vi "process_stim_NI.vi"(8 "error in (no error)":errorcluster) -> (0 "error out":errorcluster)   [LabVIEW 2010]
uses:
  typedefs/control_stim_enum.ctl
  typedefs/run_mode.ctl
  typedefs/device_parameters.ctl
  typedefs/protocol_parameters.ctl
  typedefs/free_run_parameters.ctl
  <vilib>/DAQmx/write.llb/DAQmx Write (Analog 1D DBL 1Chan NSamp).vi
  <vilib>/daqmx/miscellaneous.llb/DAQmx Fill In Error Info.vi
  Program Files/National Instruments/LabVIEW 2010/resource/objmgr/daqmx.rc
panel:
  out "Time [s]":dbl caption="[s]"
  out "Protocol":dbl[](graph)
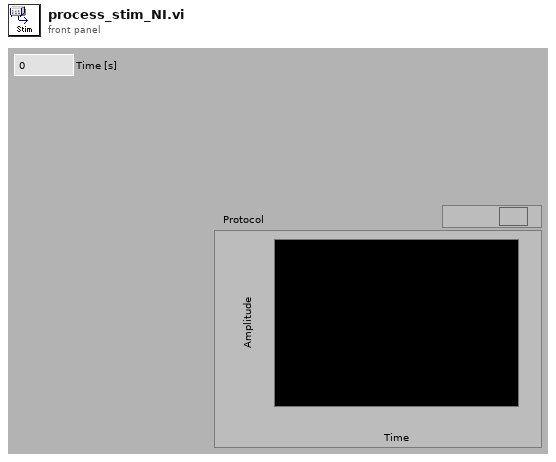
[diagram p1: front panel]
types:
  T1 = typedef "control_stim_enum.ctl" = enum16{"Init", "Stim Protocol", "Stim Free Run", "Stop", "Quit"}
  T2 = cluster{"Control stim Enum":T1, "variant":variant}
  T3 = typedef "run_mode.ctl" = enum32{"Protocol", "Free Run"}
  T4 = typedef "device_parameters.ctl" = cluster{"Triggered?":bool, "Shutter channel":tag, "Acquisition channels":tag, "Acquisition sample rate":dbl, "Read chunk size":i32, "Stimulation channel":tag, "Stimulation sample rate":dbl}
  T5 = typedef "protocol_parameters.ctl" = cluster{"Repetitions":dbl, "ON time":dbl, "OFF time":dbl, "Stim onset":dbl, "Stim frequency":dbl, "Pulse width":dbl, "Acquire before ON":dbl, "Acquire after ON":dbl, "Sync shutter to acquisition":bool}
  T6 = cluster{"Device parameters":T4, "Protocol parameters":T5}
  T7 = typedef "free_run_parameters.ctl" = cluster{"Stim onset":dbl, "Stim frequency":dbl, "Stim length":dbl, "Sync shutter to acquisition":bool}
  T8 = cluster{"Device parameters":T4, "Free run parameters":T7}
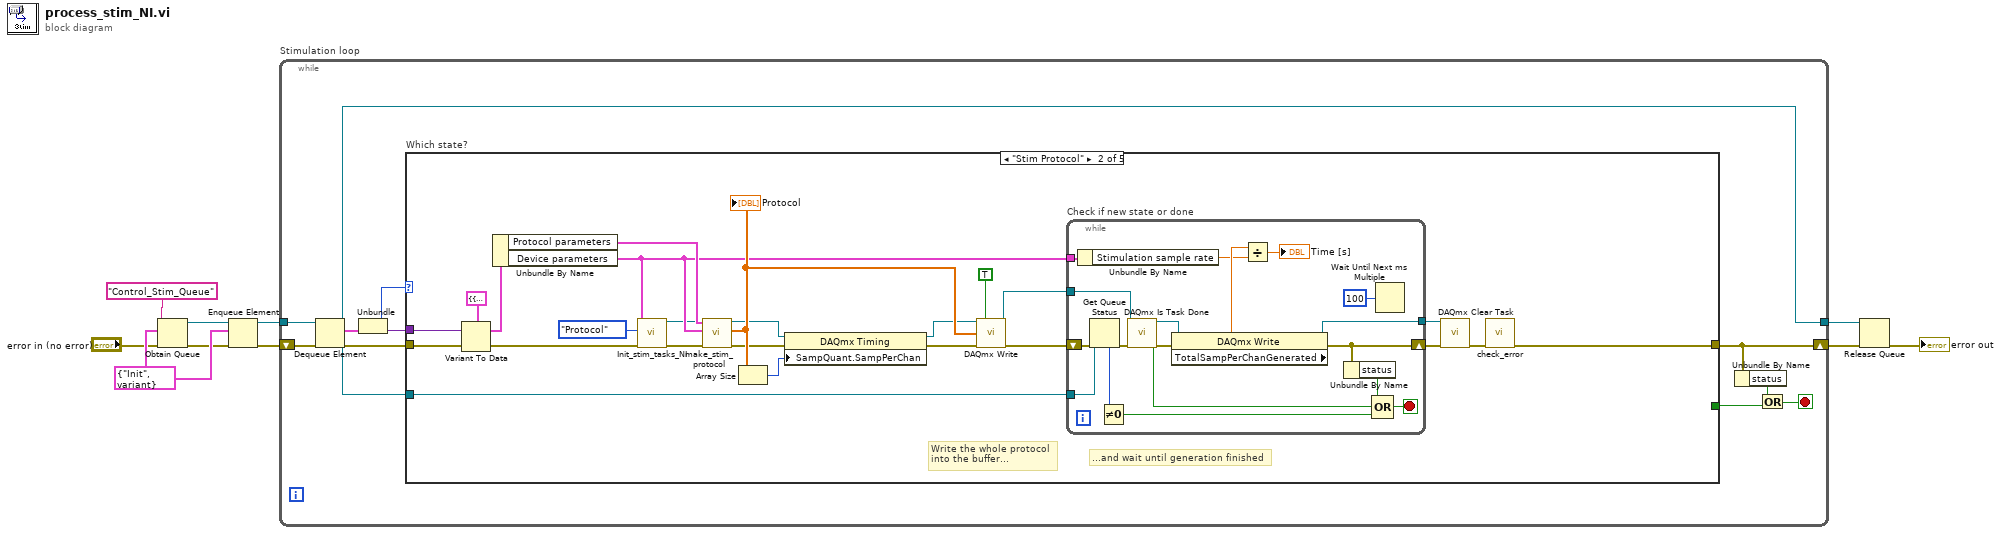
[diagram p0: block diagram]
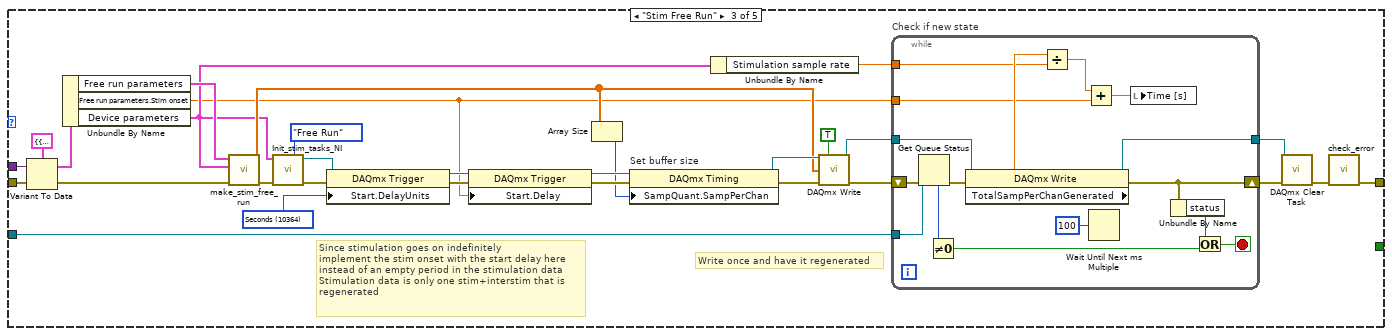
[diagram p3: hidden frame]
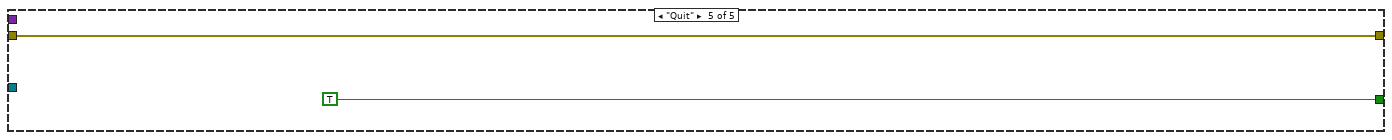
[diagram p5: hidden frame]
diagram:
  w10 = T2 {"Control stim Enum"=enum."Init", "variant"=variant} ("ControlDAQ state cluster")
  n1 = Obtain Queue(name (unnamed)="Control_Stim_Queue", element data type=w10, error in (no error)="error in (no error)") -> (queue out=w6:refnum<queue>, error out=w8:errorcluster)  [unwired: 2 in, 1 out]
  n2 = Enqueue Element(queue=w6, element=w10, error in (no error)=w8) -> (queue out=w7:refnum<queue>, error out=w9:errorcluster)  [unwired: 1 in, 1 out]
  n3 = while "Stimulation loop" {
    shift-right: [w15] -> w5
    shift-left: w9 -> [w20]
    tunnel: w7 -> [w21]
    tunnel: [w11] -> w4
    stop <- w13 stop-if-true
    n4 = Dequeue Element(queue=w21, error in (no error)=w20) -> (queue out=w11:refnum<queue>, element=w19:T2, error out=w17:errorcluster)  [unwired: 1 in, 1 out]
    n5 = Unbundle(w19) -> ("Control stim Enum"=w12:T1, "variant"=w18:variant)
    n6 = case "Which state?" shown="\"Stim Protocol\"" w12 {
      tunnel: w11 -> [_ w43 w72 _ _]
      tunnel: w18 -> [_ w45 w92 _ _]
      tunnel: w17 -> [w22 w44 w93 w110 w111]
      tunnel: [w22 w29 w67 w110 w111] -> w15
      tunnel: [_ _ _ _ TRUE] -> w16
      frame "Init", Default {
      }
      frame "Stim Protocol" {
        # "...and wait until generation finished"
        # "Write the whole protocol\ninto the buffer..."
        n7 = Variant To Data(error in=w44, Variant=w45, type=T6 {"Device parameters"={"Triggered?"=FALSE, "Shutter channel"="", "Acquisition channels"="", "Acquisition sample rate"=0.0, "Read chunk size"=0, "Stimulation channel"="", "Stimulation sample rate"=0.0}, "Protocol parameters"={"Repetitions"=0.0, "ON time"=0.0, "OFF time"=0.0, "Stim onset"=0.0, "Stim frequency"=0.0, "Pulse width"=0.0, "Acquire before ON"=0.0, "Acquire after ON"=0.0, "Sync shutter to acquisition"=FALSE}}) -> (error out=w42:errorcluster, data=w39:T6)
        n8 = Unbundle By Name(w39) -> ("Protocol parameters"=w38:T5, "Device parameters"=w28:T4)
        n9 = call "Init_stim_tasks_NI.vi"("error in"=w42, "Run mode"=run_mode."Protocol", "Device parameters"=w28) -> ("error out"=w41:errorcluster, "Stim task out"=w27:refnum<k21>)  [unwired: 5 in]
        n10 = call "make_stim_protocol.vi"("Error in"=w41, "Device parameters"=w28, "Protocol parameters"=w38) -> ("Error out"=w24:errorcluster, "Stim array"=w37:dbl[])  [unwired: 7 in]
        "Protocol" <- w37
        n11 = Array Size(array=w37) -> (size(s)=w23:i32)
        n12 = property class="DAQmx Timing"(reference=w27, error in=w24, "SampQuant.SampPerChan"=w23) -> (reference out=w26:refnum<k21>, error out=w25:errorcluster)
        n13 = call-poly <vilib>:"DAQmx Write.vi"("task/channels in"=w26, "auto start"=TRUE, "data"=w37, "error in"=w25) -> ("task out"=w34:refnum<k21>, "error out"=w35:errorcluster)  [unwired: 9 in, 1 out]
        n14 = while "Check if new state or done" {
          tunnel: w43 -> [w63]
          tunnel: w34 -> [w60]
          tunnel: [w50] -> w33
          shift-right: [w52] -> w32
          shift-left: w35 -> [w62]
          tunnel: w28 -> [w49]
          stop <- w54 stop-if-true
          n15 = Unbundle By Name(w49) -> ("Stimulation sample rate"=w47:dbl)
          n16 = Get Queue Status(queue=w63, error in (no error)=w62) -> (error out=w61:errorcluster, # elements in queue=w59:i32)  [unwired: 1 in, 6 out]
          n17 = Not Equal To 0?(x=w59) -> (x != 0?=w55:bool)
          n18 = call <vilib>:"DAQmx Is Task Done.vi"("task/channels in"=w60, "error in"=w61) -> ("task out"=w51:refnum<k21>, "task done?"=w56:bool, "error out"=w53:errorcluster)  [unwired: 11 in]
          n19 = property class="DAQmx Write"(reference=w51, error in=w53) -> (reference out=w50:refnum<k21>, error out=w52:errorcluster, "TotalSampPerChanGenerated"=w48:dbl)
          n20 = Divide(x=w48, y=w47) -> (x/y=→"Time [s]":dbl)
          n21 = Unbundle By Name(w52) -> ("status"=w57:bool)
          n22 = Compound Arithmetic op=OR(w57, w56, w55) -> (w54:bool)
          n23 = Wait Until Next ms Multiple(millisecond multiple=u32 100) -> ()  [unwired: 1 out]
        }
        n24 = call <vilib>:"DAQmx Clear Task.vi"("task in"=w33, "error in"=w32) -> ("error out"=w30:errorcluster)  [unwired: 13 in]
        n25 = call "check_error.vi"("error in"=w30) -> ("error out"=w29:errorcluster)  [unwired: 10 in]
      }
      frame "Stim Free Run" {
        w87 = 10364 items=["Sample Clock Periods"=10286, "Seconds"=10364, "Ticks"=10304] ("Start.DelayUnits")
        # "Write once and have it regenerated"
        # "Since stimulation goes on indefinitely\nimplement the stim onset with the start delay here\ninstead of an empty period in the stimulation data\nStimulation data is only one stim+interstim that is\nregenerated"
        n26 = Variant To Data(error in=w93, Variant=w92, type=T8 {"Device parameters"={"Triggered?"=FALSE, "Shutter channel"="", "Acquisition channels"="", "Acquisition sample rate"=0.0, "Read chunk size"=0, "Stimulation channel"="", "Stimulation sample rate"=0.0}, "Free run parameters"={"Stim onset"=0.0, "Stim frequency"=0.0, "Stim length"=0.0, "Sync shutter to acquisition"=FALSE}} ("output cluster")) -> (error out=w82:errorcluster, data=w90:T8)
        n27 = Unbundle By Name(w90) -> ("Free run parameters"=w83:T7, "Free run parameters.Stim onset"=w64:dbl, "Device parameters"=w66:T4)
        n28 = call "make_stim_free_run.vi"("error in"=w82, "Device parameters"=w66, "Free run parameters"=w83) -> ("error out"=w81:errorcluster, "Stim array"=w75:dbl[])  [unwired: 7 in]
        n29 = call "Init_stim_tasks_NI.vi"("error in"=w81, "Run mode"=run_mode."Free Run", "Device parameters"=w66) -> ("error out"=w85:errorcluster, "Stim task out"=w84:refnum<k21>)  [unwired: 5 in]
        n30 = property class="DAQmx Trigger"(reference=w84, error in=w85, "Start.DelayUnits"=w87) -> (reference out=w88:refnum<k21>, error out=w89:errorcluster)
        n31 = property class="DAQmx Trigger"(reference=w88, error in=w89, "Start.Delay"=w64) -> (reference out=w79:refnum<k21>, error out=w80:errorcluster)
        n32 = Array Size(array=w75) -> (size(s)=w78:i32)
        n33 = property on="Set buffer size" class="DAQmx Timing"(reference=w79, error in=w80, "SampQuant.SampPerChan"=w78) -> (reference out=w76:refnum<k21>, error out=w77:errorcluster)
        n34 = Unbundle By Name(w66) -> ("Stimulation sample rate"=w65:dbl)
        n35 = call-poly <vilib>:"DAQmx Write.vi"("task/channels in"=w76, "auto start"=TRUE, "data"=w75, "error in"=w77) -> ("task out"=w69:refnum<k21>, "error out"=w73:errorcluster)  [unwired: 9 in, 1 out]
        n36 = while "Check if new state" {
          tunnel: w72 -> [w108]
          shift-right: [w101] -> w71
          shift-left: w73 -> [w109]
          tunnel: w69 -> [w98]
          tunnel: [w97] -> w70
          tunnel: w65 -> [w99]
          tunnel: w64 -> [w96]
          stop <- w104 stop-if-true
          n37 = Get Queue Status(queue=w108, error in (no error)=w109) -> (error out=w102:errorcluster, # elements in queue=w107:i32)  [unwired: 1 in, 6 out]
          n38 = Not Equal To 0?(x=w107) -> (x != 0?=w106:bool)
          n39 = property class="DAQmx Write"(reference=w98, error in=w102) -> (reference out=w97:refnum<k21>, error out=w101:errorcluster, "TotalSampPerChanGenerated"=w100:dbl)
          n40 = Divide(x=w100, y=w99) -> (x/y=w95:dbl)
          n41 = Add(x=w95, y=w96) -> (x+y=w94:dbl)
          n42 = Wait Until Next ms Multiple(millisecond multiple=u32 100) -> ()  [unwired: 1 out]
          n43 = local write "Time [s]"(w94) -> ()
          n44 = Unbundle By Name(w101) -> ("status"=w105:bool)
          n45 = Or(x=w105, y=w106) -> (x .or. y?=w104:bool)
        }
        n46 = call <vilib>:"DAQmx Clear Task.vi"("task in"=w70, "error in"=w71) -> ("error out"=w68:errorcluster)  [unwired: 13 in]
        n47 = call "check_error.vi"("error in"=w68) -> ("error out"=w67:errorcluster)  [unwired: 10 in]
      }
      frame "Stop" {
      }
      frame "Quit" {
      }
    }
    n48 = Unbundle By Name(w15) -> ("status"=w14:bool)
    n49 = Or(x=w14, y=w16) -> (x .or. y?=w13:bool)
  }
  n50 = Release Queue(queue=w4, error in (no error)=w5) -> (error out=→"error out":errorcluster)  [unwired: 1 in, 2 out]
